vi "test - Auto Removal of Rules in CSM.vi"(8 "error in (no error)":errorcluster, 11 "TestCase in":refnum<class "testcase-Broadcast Registry.lvclass">) -> (0 "error out":errorcluster, 3 "TestCase out":refnum<class "testcase-Broadcast Registry.lvclass">)   [LabVIEW 2017, in "testcase-Broadcast Registry.lvclass"]
uses:
  testcase-Broadcast Registry.lvclass
  f1ab6f25-c30d-499f-96ca-3a55fa643449.vi
  3333bc11-4669-4098-bb8f-070e1dff9beb.vi
  src/user.lib/_NEVSTOP/Communicable State Machine(CSM)/AdvanceAPI/CSM - Revert Arguments-Safe String.vi
  src/user.lib/_NEVSTOP/Communicable State Machine(CSM)/AdvanceAPI/CSM - Make String Arguments Safe.vi
  src/user.lib/_NEVSTOP/Communicable State Machine(CSM)/AdvanceAPI/CSM - Break Down Multiple States String.vi
  src/user.lib/_NEVSTOP/Communicable State Machine(CSM)/AdvanceAPI/CSM - Compact Multiple States.vi
  src/user.lib/_NEVSTOP/Communicable State Machine(CSM)/AdvanceAPI/CSM - Keywords.vi
  src/user.lib/_NEVSTOP/Communicable State Machine(CSM)/_Shared/Trim Single-line Text.vi
  <vilib>/addons/_JKI Toolkits/VI Tester/TestCase.llb/TestCase.lvclass
  src/user.lib/_NEVSTOP/Communicable State Machine(CSM)/Communicable State Machine.lvlib
  C:/Program Files (x86)/National Instruments/LabVIEW 2017/vi.lib/addons/_JKI Toolkits/VI Tester/TestCase.llb/TestCase.lvclass
panel:
  out "Entries":T1(array[cluster])
  out "Error Occurred":errorcluster
  out "State History":string
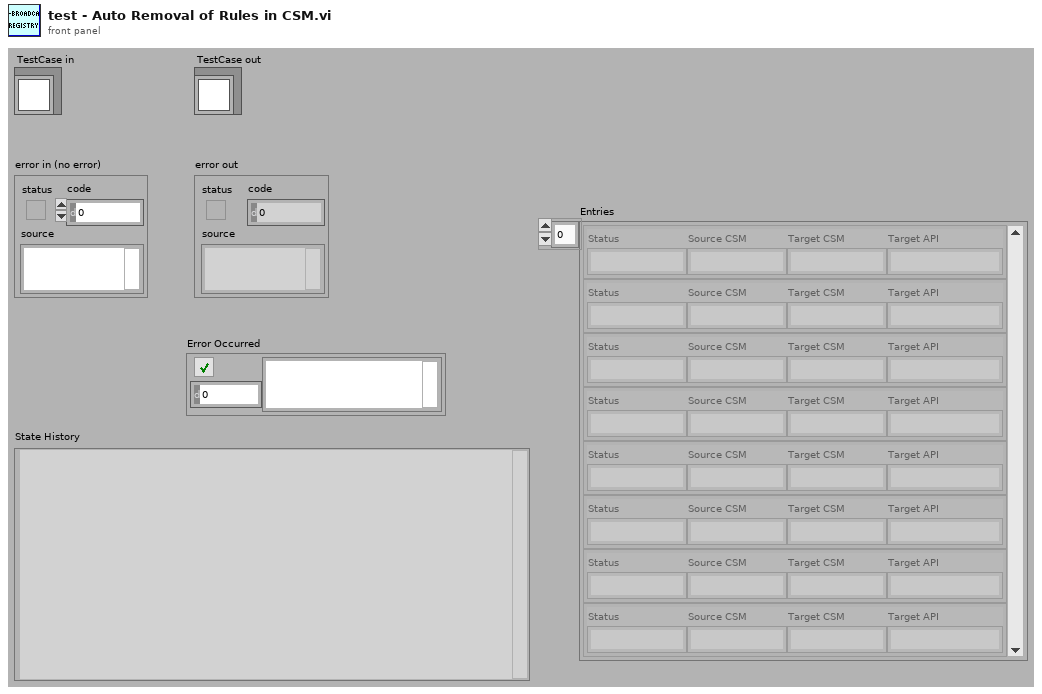
[diagram p1: front panel]
types:
  T1 = cluster{"Status":string, "Source CSM":string, "Target CSM":string, "Target API":string}[]
  T2 = enum32{"Invalid", "Standard", "Closed", "Hidden", "Minimized", "Maximized"}
  T3 = enum32{"invalid app kind", "Development System", "Run Time System", "Student Edition", "Embedded LabVIEW", "Evaluation", "Custom"}
  T4 = typedef "Communicable State Machine.lvlib/_CSM_Response Source Message.ctl" = cluster{"‘State":string, "’Arguments":string, "’Error":errorcluster}
  T5 = cluster{"Current VI Reference":refnum<vi>, "Close Panel on Exit?":bool}
  T6 = cluster{"Core":cluster{"Current VI Reference":refnum<vi>, "Close Panel on Exit?":bool}, "Your Boolean data":bool, "Your string data":string}
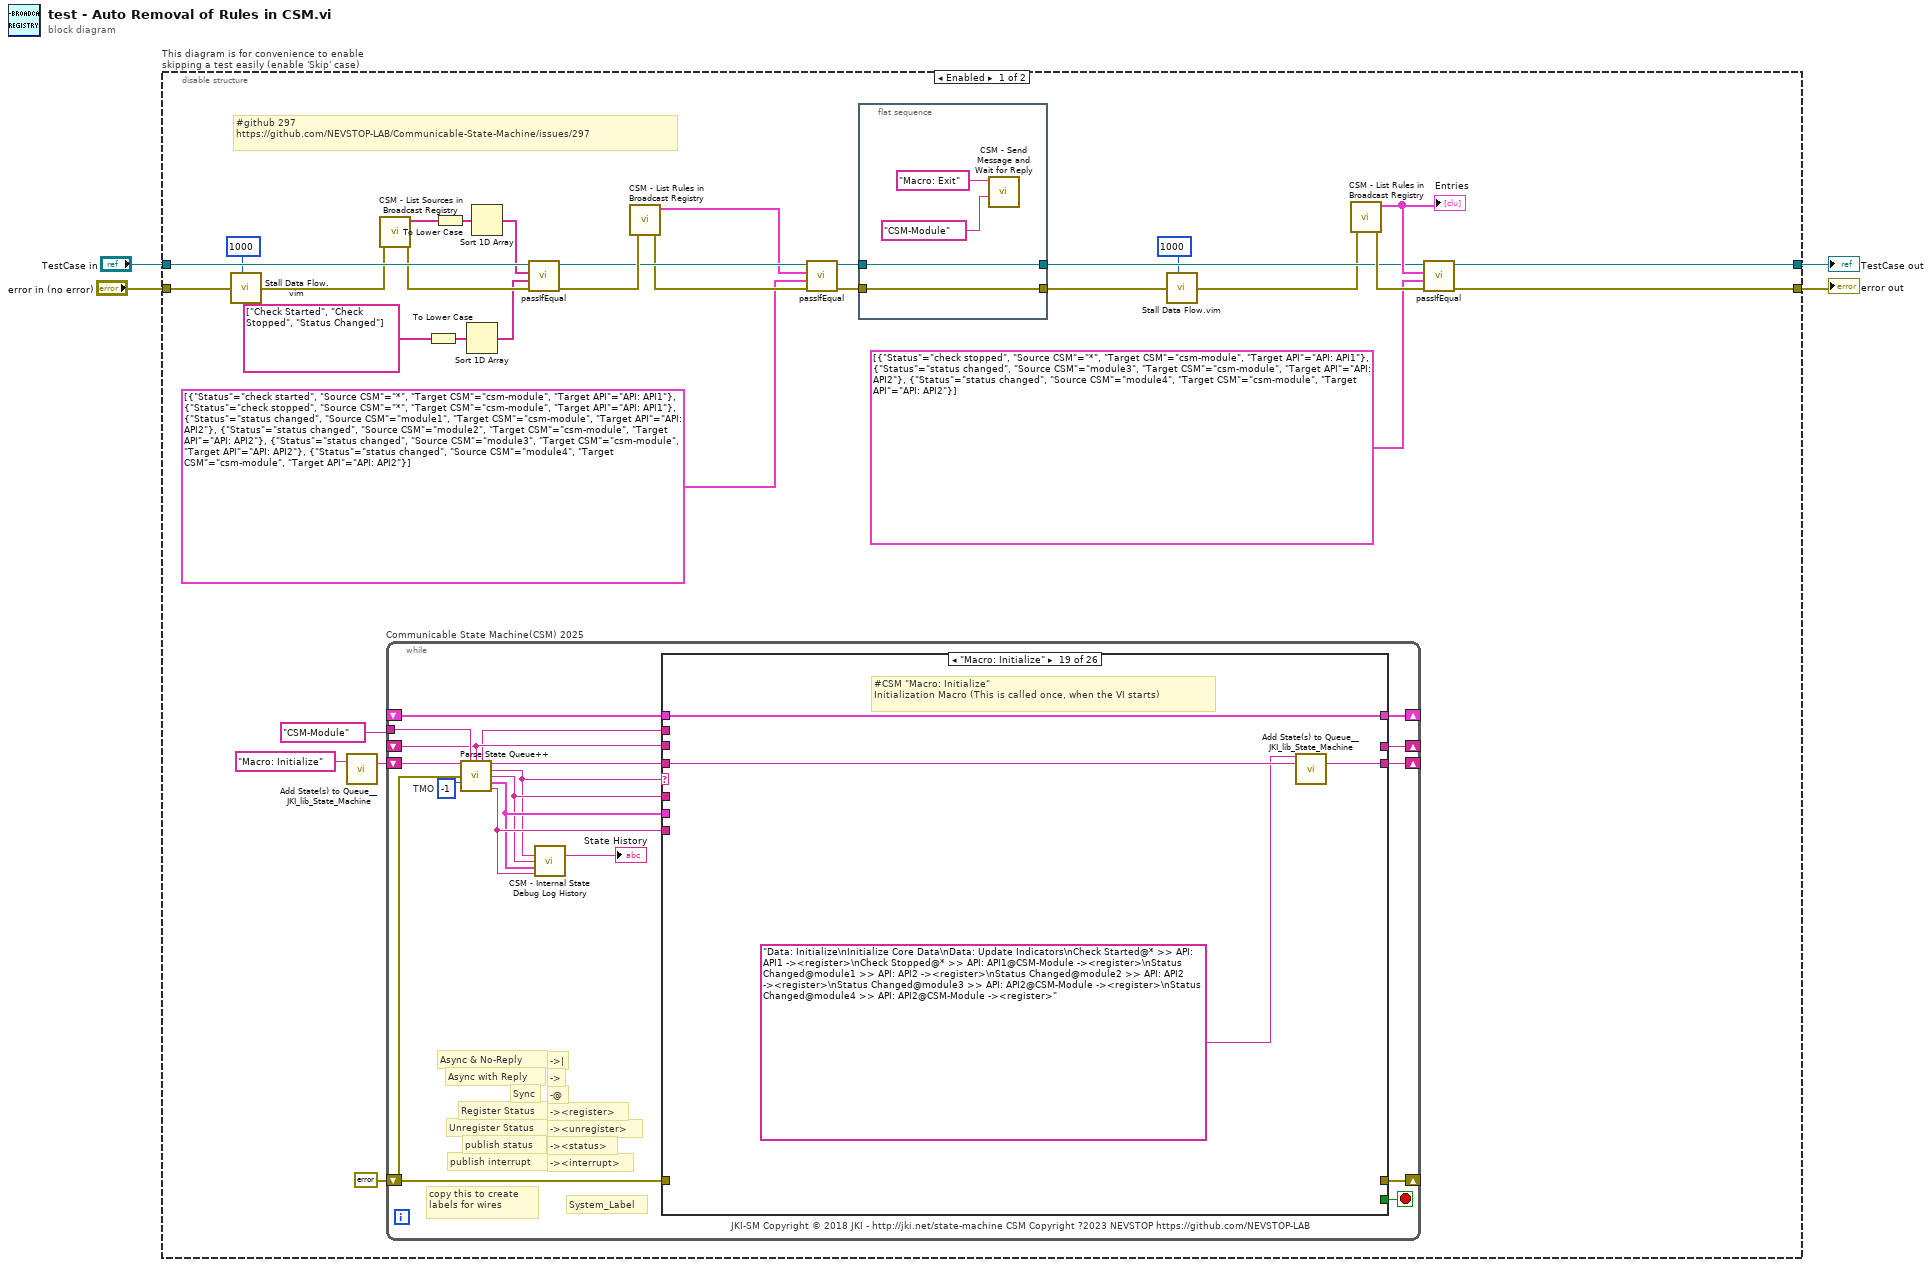
[diagram p0: block diagram]
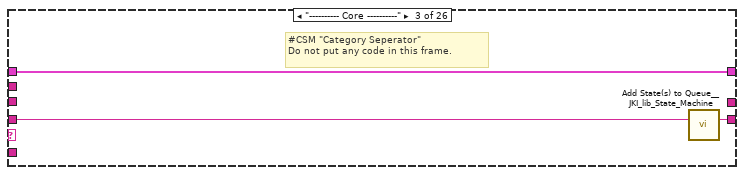
[diagram p4: hidden frame]
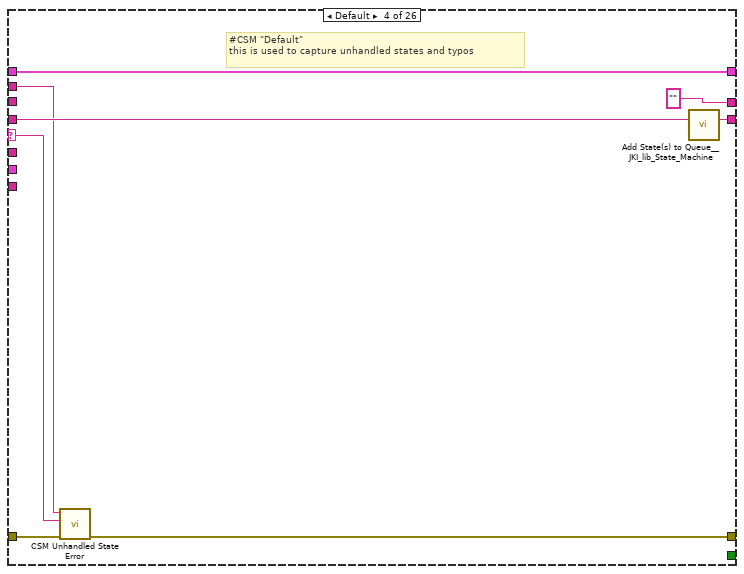
[diagram p5: hidden frame]
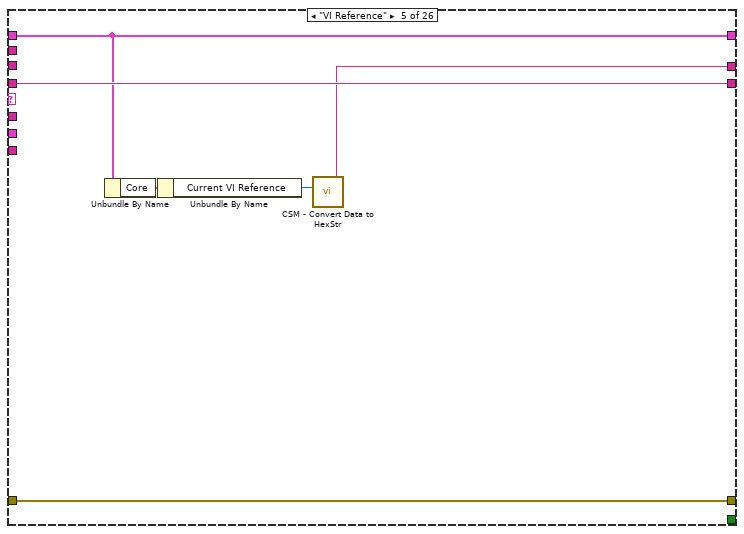
[diagram p6: hidden frame]
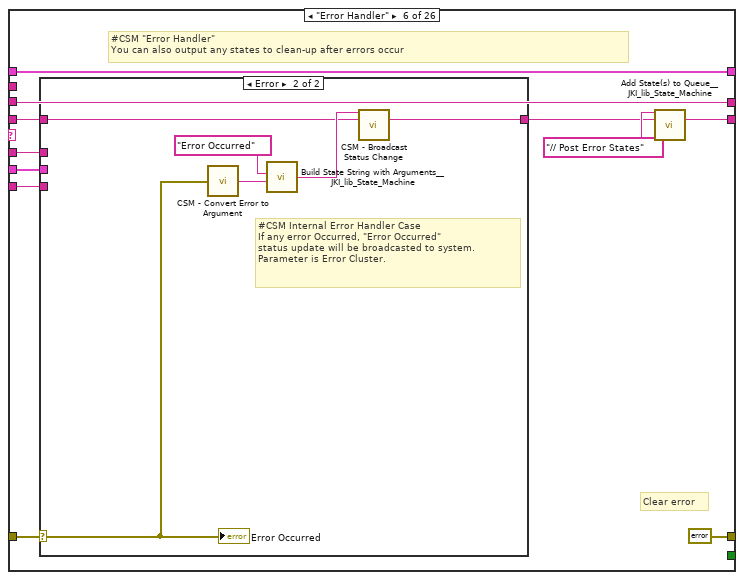
[diagram p7: hidden frame]
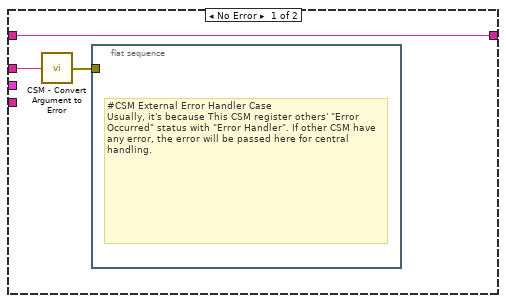
[diagram p8: hidden frame]
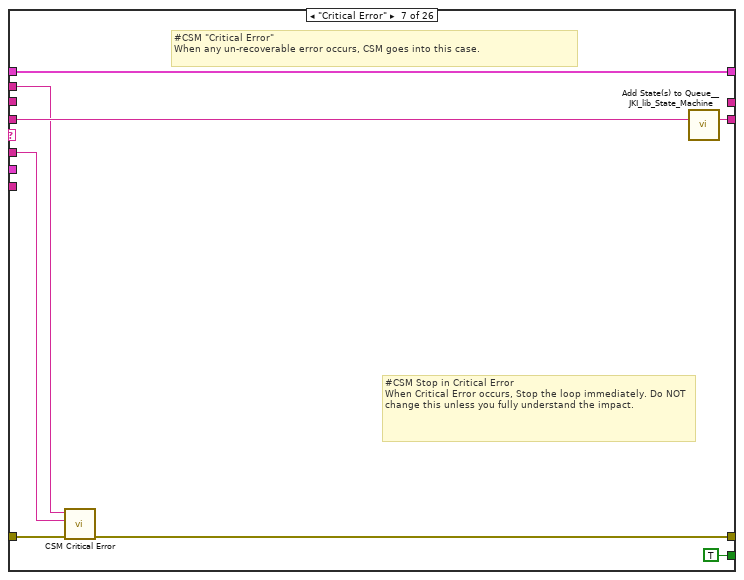
[diagram p9: hidden frame]
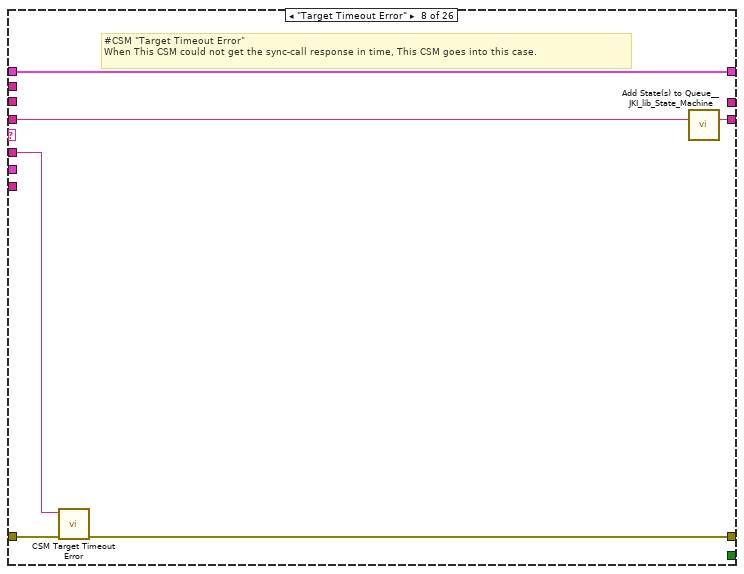
[diagram p10: hidden frame]
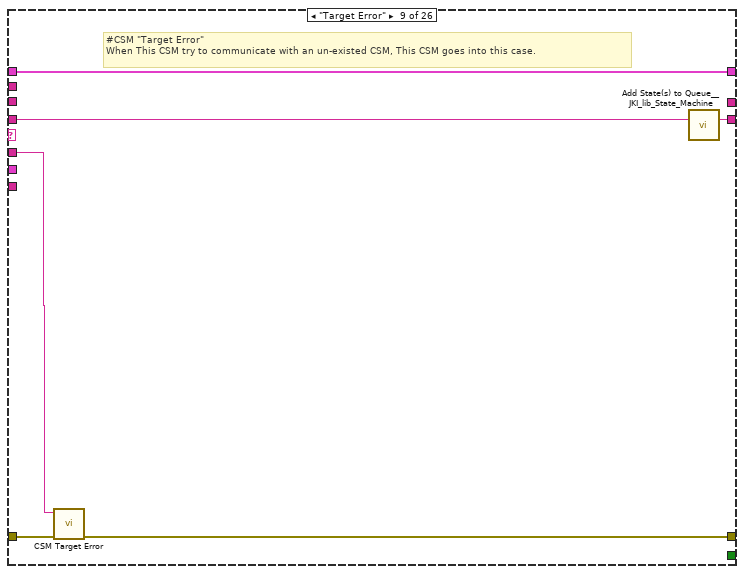
[diagram p11: hidden frame]
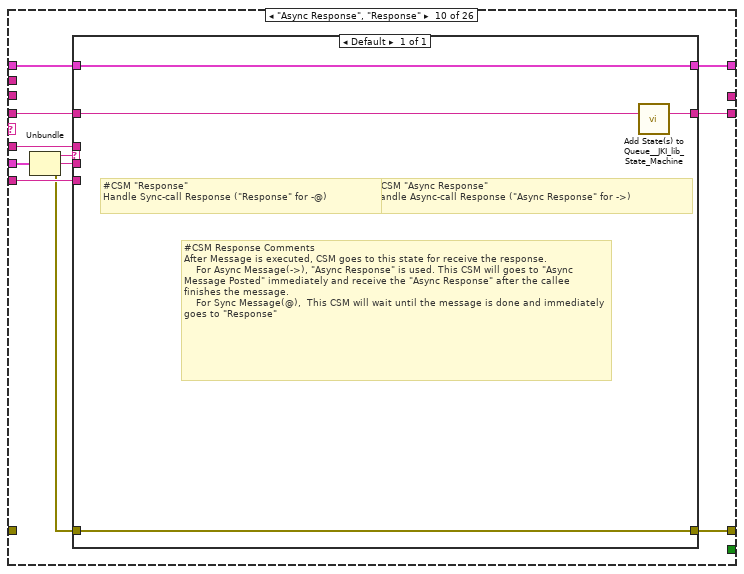
[diagram p12: hidden frame]
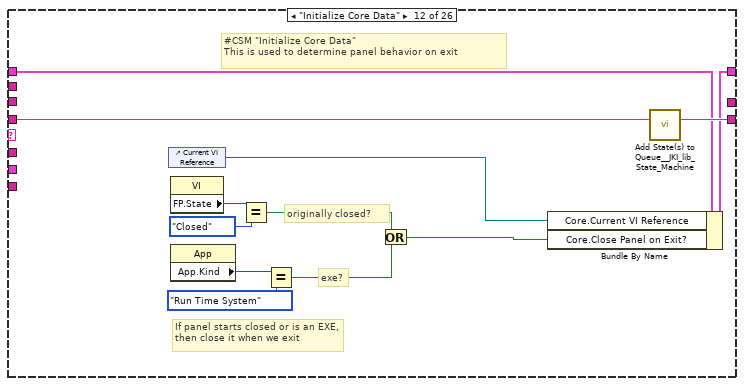
[diagram p14: hidden frame]
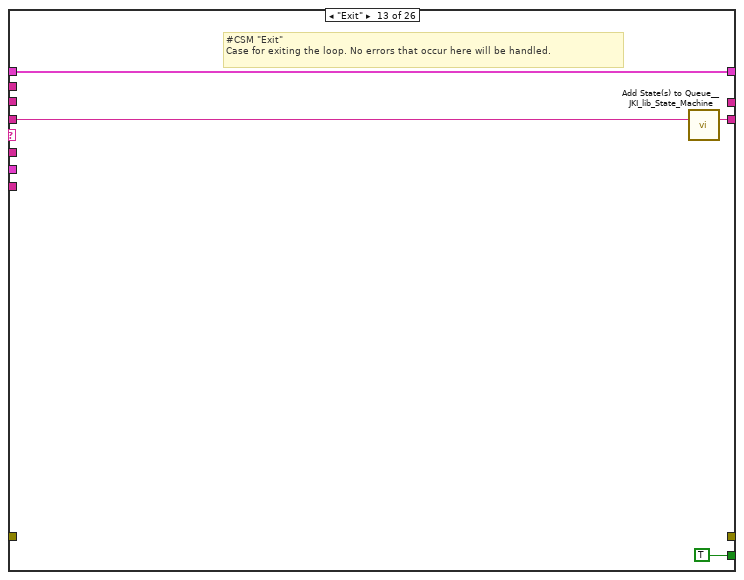
[diagram p15: hidden frame]
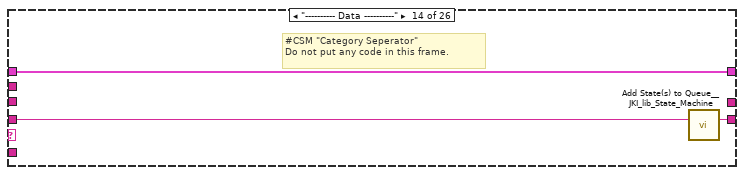
[diagram p16: hidden frame]
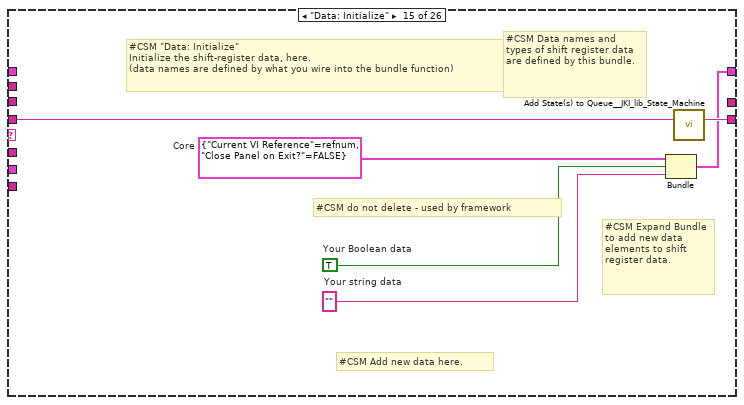
[diagram p17: hidden frame]
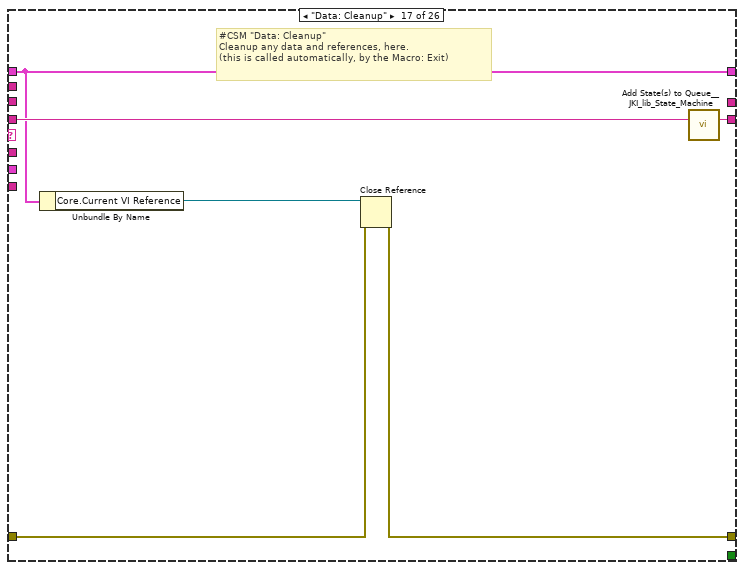
[diagram p19: hidden frame]
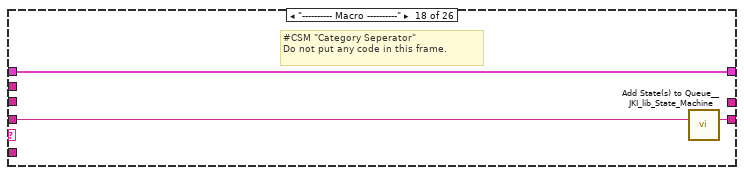
[diagram p20: hidden frame]
diagram:
  n1 = disable-structure "This diagram is for convenience to enable skipping a test easily (enable 'Skip' case)" shown="Enabled" {
    disable-tunnel: "TestCase in" -> [w35 w205]
    disable-tunnel: [w17 w203] -> w1
    disable-tunnel: [w24 w204] -> w3
    disable-tunnel: "error in (no error)" -> [w34 w202]
    frame Enabled {
      # "#github 297\nhttps://github.com/NEVSTOP-LAB/Communicable-State-Machine/issues/297"
      n2 = call "Stall Data Flow.vim"("value in"=w34, "milliseconds to wait"=u32 1000) -> ("value out"=w29:errorcluster)  [unwired: 1 out]
      n3 = call <vilib>:"Add State(s) to Queue__JKI_lib_State_Machine.vi"("State(s) in (\"\")"="Macro: Initialize" ("Init State(\"Macro: Initialize\")")) -> ("States Out"=w33:string)  [unwired: 14 in]
      n4 = call "CSM - List Sources in Broadcast Registry.vi"("error in (no error)"=w29) -> ("error out"=w27:errorcluster, "Broadcast Names"=w26:string[])  [unwired: 9 in]
      n5 = while "Communicable State Machine(CSM) 2025" {
        shift-right: [w52] -> _
        shift-left: _ -> [w51]
        shift-right: [w55] -> _
        shift-left: errorcluster {"status"=FALSE, "code"=0, "source"=""} ("error out") -> [w41]
        shift-right: [w54] -> _
        shift-left: w33 -> [w56]
        tunnel: "CSM-Module" ("Name (\"\" to Use UUID)") -> [w48]
        shift-right: [w49] -> _
        shift-left: _ -> [w43]
        stop <- w53 stop-if-true
        w50 = -1  # TMO
        # "-><interrupt>"
        # "-><status>"
        # "-><unregister>"
        # "-><register>"
        # "-@"
        # "->"
        # "->|"
        # "publish interrupt"
        # "publish status"
        # "Unregister Status"
        # "Register Status"
        # "Sync"
        # "Async with Reply"
        # "Async & No-Reply"
        # "JKI-SM Copyright © 2018 JKI - http://jki.net/state-machine CSM Copyright ?2023 NEVSTOP https://github.com/NEVSTOP-LAB"
        # "copy this to create labels for wires"
        # "System_Label"
        n6 = call "Parse State Queue++.vi"("State Queue"=w56, "Name (\"\" to Use UUID)"=w48, "Response Arguments"=w43, "Previous Error"=w41, "Dequeue (1 ms)"=w50) -> ("Name Used"=w42:string, "Remaining States"=w57:string, "Current State"=w44:string, "Arguments"=w45:string, "Additional Information"=w46:T4, "Source CSM"=w47:string)  [unwired: 5 in]
        n7 = call "CSM - Internal State Debug Log History.vi"("State"=w44, "Arguments (\"\")"=w45, ">> Response Source Message >>"=w46, "Source (\"\")"=w47) -> ("Debug Log"=→"State History":string)  [unwired: 11 in]
        n8 = case shown="\"Macro: Initialize\"" w44 {
          selector: w44 -> [_ _ _ w68 _ _ _ _ _ _ _ _ _ _ _ _ _ _ _ _ _ _ _ _ _ _]
          tunnel: w57 -> [w58 w61 w64 w72 w77 w83 w106 w112 w118 w128 w135 w147 w151 w154 w160 w162 w168 w171 w175 w181 w183 w186 w190 w195 w198 w201]
          tunnel: w45 -> [_ _ _ _ _ w82 w102 w109 w115 w122 _ _ _ _ _ _ _ _ _ _ _ _ w188 _ _ _]
          tunnel: w51 -> [w59 w60 w62 w70 w76 w88 w104 w110 w116 w126 w134 w141 w149 w152 _ w161 w163 w169 w173 w179 w182 w185 w189 w193 w196 w199]
          tunnel: [_ _ _ w65 w78 errorcluster {"status"=FALSE, "code"=0, "source"=""} ("error out") w99 w107 w113 w129 _ _ _ _ _ _ w164 _ _ _ _ _ _ _ _ _] -> w55
          tunnel: w41 -> [_ _ _ w66 w78 w86 w100 w108 w114 _ _ _ _ _ _ _ w165 _ _ _ _ _ _ _ _ _]
          tunnel: [w58 w61 w63 w71 w77 w84 w105 w111 w117 w127 w135 w146 w150 w153 w159 w162 w167 w170 w174 w180 w183 w186 w190 w194 w197 w200] -> w54
          tunnel: [_ _ _ _ _ _ TRUE _ _ _ _ _ TRUE _ _ _ _ _ _ _ _ _ _ _ _ _] -> w53
          tunnel: [w59 w60 w62 w70 w76 w88 w104 w110 w116 w125 w134 w145 w149 w152 w158 w161 w163 w169 w173 w179 w182 w185 w189 w193 w196 w199] -> w52
          tunnel: w47 -> [_ _ _ _ _ w81 _ _ _ w123 _ _ _ _ _ _ _ _ _ _ _ _ _ _ _ _]
          tunnel: w46 -> [_ _ _ _ _ w80 _ _ _ w124 _ _ _ _ _ _ _ _ _ _ _ _ _ _ _ _]
          tunnel: [_ _ _ "" w73 w79 _ _ _ _ _ _ _ _ _ _ _ _ _ _ _ "API1 Response" w187 _ _ _] -> w49
          tunnel: w42 -> [_ _ _ w67 _ _ w101 _ _ _ _ _ _ _ _ _ _ _ _ _ _ _ _ _ _ _]
          tunnel: w43 -> [_ _ _ _ _ w79 _ _ _ _ _ _ _ _ _ _ _ _ _ _ _ _ _ _ _ _]
          frame "", "Idle" {
            # "#CSM \"Idle/Event Handler\"\nexecutes when the state queue is empty"
          }
          frame "CSM Documentation" {
            # "#CSM Documentation"
            # "#CSM State Syntax\n\n// Comment line, all text to the right of “//” will be ignored\n// Local Message Example\nDoSth: DoA >> Arguments\n\n// Sync Call Example\nAPI: xxxx >> Arguments -@ TargetModule\n\n// Async Call Example\nAPI: xxxx >> Arguments -> TargetModule\n\n// Async Call without Reply Example\nAPI: xxxx >> Arguments ->| TargetModule\n\n// Broadcast normal status:\nStatus >> StatusArguments  -><status>\n\n// Broadcast Interrupt status:\nInterrupt >> StatusArguments  -><interrupt>\n\n// Register Source Module's status to Handler Module\nStatus@Source Module >> Handler Module@Handler Module -><register>\n\n// Unegister Source Module's status\nStatus@Source Module >> Handler Module -><unregister>"
            # "#CSM README FIRST\n\nCommunicable State Machine(CSM) is a LabVIEW application framework that builds upon JKI State Machine(JKISM). It follows the pattern of JKISM and extends the keywords to describe message communication between modules, including concepts such as Sync-Message, Async-Message, Subscription/Unsubscription of status - essential elements for creating reusable code modules. For more information, please visit the CSM wiki: https://nevstop-lab.github.io/CSM-Wiki/\n\nFor instructions on JKI State Machine, visit: \n    http://jki.net/state-machine/\nFor information about CSM, visit: \n    https://github.com/NEVSTOP-LAB"
            # "#CSM \"Documentation\"\nCase for holding CSM Documenation"
          }
          frame "---------- Core ----------" {
            # "#CSM \"Category Seperator\"\nDo not put any code in this frame."
            n9 = call <vilib>:"Add State(s) to Queue__JKI_lib_State_Machine.vi"("State(s) in (\"\")"=w64) -> ("States Out"=w63:string)  [unwired: 14 in]
          }
          frame Default {
            # "#CSM \"Default\"\nthis is used to capture unhandled states and typos"
            n10 = call "CSM Unhandled State Error.vi"("error in (no error)"=w66, "Undefined State"=w68, "CSM Name"=w67) -> ("error out"=w65:errorcluster)  [unwired: 8 in]
            n11 = call <vilib>:"Add State(s) to Queue__JKI_lib_State_Machine.vi"("State(s) in (\"\")"=w72) -> ("States Out"=w71:string)  [unwired: 14 in]
          }
          frame "VI Reference" {
            n12 = Unbundle By Name(w76) -> ("Core"=w75:T5)
            n13 = Unbundle By Name(w75) -> ("Current VI Reference"=w74:refnum<vi>)
            n14 = call "CSM - Convert Data to HexStr.vi"("Variant"=w74) -> ("HEX String (0-9,A-F)"=w73:string)  [unwired: 8 in]
          }
          frame "Error Handler" {
            # "#CSM \"Error Handler\"\nYou can also output any states to clean-up after errors occur"
            # "Clear error"
            n15 = case shown="Error" w86 {
              selector: w86 -> [_ w93]
              tunnel: [w92 w95] -> w85
              tunnel: w83 -> [w92 w94]
              tunnel: w82 -> [w91 _]
              tunnel: w81 -> [_ _]
              tunnel: w80 -> [_ _]
              frame No Error {
                n16 = call "CSM - Convert Argument to Error.vi"("Argument"=w91) -> ("Error"=w90:errorcluster)  [unwired: 4 in]
                n17 = flat-sequence {
                  tunnel: w90 -> [_]
                  frame #0 {
                    # "#CSM External Error Handler Case\nUsually, it's because This CSM register others' \"Error Occurred\" status with \"Error Handler\". If other CSM have any error, the error will be passed here for central handling."
                  }
                }
              }
              frame Error {
                # "#CSM Internal Error Handler Case \nIf any error Occurred, \"Error Occurred\" \nstatus update will be broadcasted to system.\nParameter is Error Cluster."
                n18 = call "CSM - Convert Error to Argument.vi"("Error"=w93) -> ("Argument"=w97:string)  [unwired: 4 in]
                n19 = call <vilib>:"Build State String with Arguments__JKI_lib_State_Machine.vi"("Arguments (\"\")"=w97, "State"="Error Occurred" ("Status with Arguments")) -> ("State with Arguments"=w96:string)  [unwired: 4 in]
                n20 = call "CSM - Broadcast Status Change.vi"("Status With Arguments"=w96, "State Queue"=w94) -> ("Remaining States"=w95:string)  [unwired: 13 in]
                "Error Occurred" <- w93
              }
            }
            n21 = call <vilib>:"Add State(s) to Queue__JKI_lib_State_Machine.vi"("State(s) in Front (\"\")"="// Post Error States", "State(s) in (\"\")"=w85) -> ("States Out"=w84:string)  [unwired: 13 in]
          }
          frame "Critical Error" {
            # "#CSM \"Critical Error\"\nWhen any un-recoverable error occurs, CSM goes into this case."
            # "#CSM Stop in Critical Error\nWhen Critical Error occurs, Stop the loop immediately. Do NOT change this unless you fully understand the impact."
            n22 = call "CSM Critical Error.vi"("error in (no error)"=w100, "Arugments (As Reason)"=w102, "CSM Name"=w101) -> ("error out"=w99:errorcluster)  [unwired: 8 in]
            n23 = call <vilib>:"Add State(s) to Queue__JKI_lib_State_Machine.vi"("State(s) in (\"\")"=w106) -> ("States Out"=w105:string)  [unwired: 14 in]
          }
          frame "Target Timeout Error" {
            # "#CSM \"Target Timeout Error\"\nWhen This CSM could not get the sync-call response in time, This CSM goes into this case."
            n24 = call "CSM Target Timeout Error.vi"("error in (no error)"=w108, "Arguments (As CSM Name)"=w109) -> ("error out"=w107:errorcluster)  [unwired: 9 in]
            n25 = call <vilib>:"Add State(s) to Queue__JKI_lib_State_Machine.vi"("State(s) in (\"\")"=w112) -> ("States Out"=w111:string)  [unwired: 14 in]
          }
          frame "Target Error" {
            # "#CSM \"Target Error\"\nWhen This CSM try to communicate with an un-existed CSM, This CSM goes into this case."
            n26 = call "CSM Target Error.vi"("error in (no error)"=w114, "Arguments (As CSM Name)"=w115) -> ("error out"=w113:errorcluster)  [unwired: 9 in]
            n27 = call <vilib>:"Add State(s) to Queue__JKI_lib_State_Machine.vi"("State(s) in (\"\")"=w118) -> ("States Out"=w117:string)  [unwired: 14 in]
          }
          frame "Async Response", "Response" {
            n28 = Unbundle(w124) -> ("‘State"=w121:string, "’Arguments"=w120:string, "’Error"=w119:errorcluster)
            n29 = case shown="Default" w121 {
              tunnel: [w130] -> w127
              tunnel: w128 -> [w131]
              tunnel: [w133] -> w125
              tunnel: w126 -> [w133]
              tunnel: [w132] -> w129
              tunnel: w119 -> [w132]
              tunnel: w123 -> [_]
              tunnel: w122 -> [_]
              tunnel: w120 -> [_]
              frame Default {
                # "#CSM \"Async Response\"\nHandle Async-call Response (\"Async Response\" for ->)"
                # "#CSM \"Response\"\nHandle Sync-call Response (\"Response\" for -@)"
                # "#CSM Response Comments\nAfter Message is executed, CSM goes to this state for receive the response.\n    For Async Message(->), \"Async Response\" is used. This CSM will goes to \"Async Message Posted\" immediately and receive the \"Async Response\" after the callee finishes the message.\n    For Sync Message(@),  This CSM will wait until the message is done and immediately goes to \"Response\""
                n30 = call <vilib>:"Add State(s) to Queue__JKI_lib_State_Machine.vi"("State(s) in (\"\")"=w131) -> ("States Out"=w130:string)  [unwired: 14 in]
              }
            }
          }
          frame "Async Message Posted" {
            # "#CSM \"Async Message Posted\"\nAfter Async Message is posted (-> or ->| ), CSM goes to this state for post-action.\nYou can use Argument - State to tell which Async Message is called."
          }
          frame "Initialize Core Data" {
            # "#CSM \"Initialize Core Data\"\nThis is used to determine panel behavior on exit"
            # "originally closed?"
            # "exe?"
            # "If panel starts closed or is an EXE, then close it when we exit"
            n31 = control-ref of="Current VI Reference"() -> (w139:refnum<vi>)
            n32 = property class="VI"() -> ("FP.State"=w138:T2)  [unwired: 2 in, 2 out]
            n33 = property class="App"() -> ("App.Kind"=w144:T3)  [unwired: 2 in, 2 out]
            n34 = Equal?(x=w138, y=T2."Closed" ("Front Panel Window:State")) -> (x = y?=w136:bool)
            n35 = Equal?(x=w144, y=T3."Run Time System" ("Application:Kind")) -> (x = y?=w142:bool)
            n36 = Or(x=w136, y=w142) -> (x .or. y?=w140:bool)
            n37 = Bundle By Name(cluster=w141, "Core.Current VI Reference"=w139, "Core.Close Panel on Exit?"=w140) -> (w145:T6)
            n38 = call <vilib>:"Add State(s) to Queue__JKI_lib_State_Machine.vi"("State(s) in (\"\")"=w147) -> ("States Out"=w146:string)  [unwired: 14 in]
          }
          frame "Exit" {
            # "#CSM \"Exit\"\nCase for exiting the loop. No errors that occur here will be handled."
            n39 = call <vilib>:"Add State(s) to Queue__JKI_lib_State_Machine.vi"("State(s) in (\"\")"=w151) -> ("States Out"=w150:string)  [unwired: 14 in]
          }
          frame "---------- Data ----------" {
            # "#CSM \"Category Seperator\"\nDo not put any code in this frame."
            n40 = call <vilib>:"Add State(s) to Queue__JKI_lib_State_Machine.vi"("State(s) in (\"\")"=w154) -> ("States Out"=w153:string)  [unwired: 14 in]
          }
          frame "Data: Initialize" {
            w155 = T5 {"Current VI Reference"=refnum, "Close Panel on Exit?"=FALSE}  # Core
            w157 = TRUE  # Your Boolean data
            w156 = ""  # Your string data
            # "#CSM \"Data: Initialize\"\nInitialize the shift-register data, here.\n(data names are defined by what you wire into the bundle function)"
            # "#CSM do not delete - used by framework"
            # "#CSM Expand Bundle to add new data elements to shift register data."
            # "#CSM Add new data here."
            # "#CSM Data names and types of shift register data are defined by this bundle."
            n41 = Bundle("Core"=w155, "Your Boolean data"=w157, "Your string data"=w156) -> (w158:T6)  [unwired: 1 in]
            n42 = call <vilib>:"Add State(s) to Queue__JKI_lib_State_Machine.vi"("State(s) in (\"\")"=w160) -> ("States Out"=w159:string)  [unwired: 14 in]
          }
          frame "Data: Update Indicators" {
          }
          frame "Data: Cleanup" {
            # "#CSM \"Data: Cleanup\"\nCleanup any data and references, here.\n(this is called automatically, by the Macro: Exit)"
            n43 = Unbundle By Name(w163) -> ("Core.Current VI Reference"=w166:refnum<vi>)
            n44 = Close Reference(reference=w166, error in (no error)=w165) -> (error out=w164:errorcluster)
            n45 = call <vilib>:"Add State(s) to Queue__JKI_lib_State_Machine.vi"("State(s) in (\"\")"=w168) -> ("States Out"=w167:string)  [unwired: 14 in]
          }
          frame "---------- Macro ----------" {
            # "#CSM \"Category Seperator\"\nDo not put any code in this frame."
            n46 = call <vilib>:"Add State(s) to Queue__JKI_lib_State_Machine.vi"("State(s) in (\"\")"=w171) -> ("States Out"=w170:string)  [unwired: 14 in]
          }
          frame "Macro: Initialize" {
            # "#CSM \"Macro: Initialize\"\nInitialization Macro (This is called once, when the VI starts)"
            n47 = call <vilib>:"Add State(s) to Queue__JKI_lib_State_Machine.vi"("State(s) in Front (\"\")"="Data: Initialize\nInitialize Core Data\nData: Update Indicators\nCheck Started@* >> API: API1 -><register>\nCheck Stopped@* >> API: API1@CSM-Module -><register>\nStatus Changed@module1 >> API: API2 -><register>\nStatus Changed@module2 >> API: API2 -><register>\nStatus Changed@module3 >> API: API2@CSM-Module -><register>\nStatus Changed@module4 >> API: API2@CSM-Module -><register>", "State(s) in (\"\")"=w175) -> ("States Out"=w174:string)  [unwired: 13 in]
          }
          frame "Macro: Exit" {
            # "#CSM \"Macro: Exit\"\nExit Macro (This is called once, when the VI exits)"
            n48 = call <vilib>:"Add State(s) to Queue__JKI_lib_State_Machine.vi"("State(s) in Front (\"\")"="//Exit Sub-Modules ", "State(s) at Back (\"\")"="Data: Cleanup\nExit") -> ("States Out"=w177:string)  [unwired: 13 in]
            n49 = call <vilib>:"Add State(s) to Queue__JKI_lib_State_Machine.vi"("State(s) in Front (\"\")"=w177, "State(s) in (\"\")"=w181) -> ("States Out"=w180:string)  [unwired: 13 in]
          }
          frame "---------- API ----------" {
            # "#CSM \"Category Seperator\"\nDo not put any code in this frame."
          }
          frame "API: API1" {
            # "#CSM API Example\nCopy/Rename this case for your own API"
            # "#CSM >> Msg/Rep's CSM >>\nIf you need to tell who triggered this state , use this string. If it's this case itself, this string is \"\"."
            # "#CSM >> Arguments >>\nDeal with the parameter if any"
            # "#CSM Response\nConnect this to return the response of your API"
          }
          frame "API: API2" {
            # "#CSM API Example\nCopy/Rename this case for your own API"
            # "unpack Hex String  to Variant\nif complex parameter is needed."
            n50 = call "CSM - Convert HexStr to Data.vi"("HEX String"=w188) -> ()  [unwired: 7 in, 2 out]
            n51 = disable-structure shown="Disabled" {
              disable-tunnel: [w191 "API2 Response"] -> w187
              frame Disabled {
                # "pack variant to hexstr \nif complex response is needed."
                # "complex Response"
                n52 = call "CSM - Convert Data to HexStr.vi"() -> ("HEX String (0-9,A-F)"=w191:string)  [unwired: 9 in]
              }
              frame Enabled {
              }
            }
          }
          frame "---------- Action ----------" {
            # "#CSM \"Category Seperator\"\nDo not put any code in this frame."
            n53 = call <vilib>:"Add State(s) to Queue__JKI_lib_State_Machine.vi"("State(s) in (\"\")"=w195) -> ("States Out"=w194:string)  [unwired: 14 in]
          }
          frame "Action: action1" {
            # "#CSM \"Internal State\"\nThis category is used for holding internal states"
            n54 = call <vilib>:"Add State(s) to Queue__JKI_lib_State_Machine.vi"("State(s) in (\"\")"=w198) -> ("States Out"=w197:string)  [unwired: 14 in]
          }
          frame "Action: action2" {
            # "#CSM \"Internal State\"\nThis category is used for holding internal states"
            n55 = call <vilib>:"Add State(s) to Queue__JKI_lib_State_Machine.vi"("State(s) in (\"\")"=w201) -> ("States Out"=w200:string)  [unwired: 14 in]
          }
        }
      }
      n56 = To Lower Case(string=string[] ["Check Started", "Check Stopped", "Status Changed"] ("Status in Registry")) -> (all lower case string=w21:string[])
      n57 = To Lower Case(string=w26) -> (all lower case string=w20:string[])
      n58 = Sort 1D Array(array=w21) -> (sorted array=w22:string[])
      n59 = Sort 1D Array(array=w20) -> (sorted array=w23:string[])
      n60 = call-dynamic "passIfEqual.vi"("error in (no error)"=w27, "y"=w22, "x"=w23, "TestCase in"=w35) -> ("error out"=w19:errorcluster, "TestCase out"=w18:refnum<class "testcase-Broadcast Registry.lvclass">)  [unwired: 6 in]
      n61 = call "CSM - List Rules in Broadcast Registry.vi"("error in (no error)"=w19) -> ("error out"=w16:errorcluster, "Rule Entries"=w15:T1)  [unwired: 9 in]
      n62 = call-dynamic "passIfEqual.vi"("error in (no error)"=w16, "y"=T1 [{"Status"="check started", "Source CSM"="*", "Target CSM"="csm-module", "Target API"="API: API1"}, {"Status"="check stopped", "Source CSM"="*", "Target CSM"="csm-module", "Target API"="API: API1"}, {"Status"="status changed", "Source CSM"="module1", "Target CSM"="csm-module", "Target API"="API: API2"}, {"Status"="status changed", "Source CSM"="module2", "Target CSM"="csm-module", "Target API"="API: API2"}, {"Status"="status changed", "Source CSM"="module3", "Target CSM"="csm-module", "Target API"="API: API2"}, {"Status"="status changed", "Source CSM"="module4", "Target CSM"="csm-module", "Target API"="API: API2"}] ("Entries"), "x"=w15, "TestCase in"=w18) -> ("error out"=w10:errorcluster, "TestCase out"=w11:refnum<class "testcase-Broadcast Registry.lvclass">)  [unwired: 6 in]
      n63 = flat-sequence {
        tunnel: [w37] -> w9
        tunnel: w10 -> [w37]
        tunnel: [w36] -> w8
        tunnel: w11 -> [w36]
        frame #0 {
          n64 = call "CSM - Send Message and Wait for Reply.vi"("Target Module"="CSM-Module" ("Name (\"\" to Use UUID)"), "State"="Macro: Exit") -> ()  [unwired: 7 in, 3 out]
        }
      }
      n65 = call "Stall Data Flow.vim"("value in"=w9, "milliseconds to wait"=u32 1000) -> ("value out"=w6:errorcluster)  [unwired: 1 out]
      n66 = call "CSM - List Rules in Broadcast Registry.vi"("error in (no error)"=w6) -> ("error out"=w14:errorcluster, "Rule Entries"=w13:T1)  [unwired: 9 in]
      "Entries" <- w13
      n67 = call-dynamic "passIfEqual.vi"("error in (no error)"=w14, "y"=T1 [{"Status"="check stopped", "Source CSM"="*", "Target CSM"="csm-module", "Target API"="API: API1"}, {"Status"="status changed", "Source CSM"="module3", "Target CSM"="csm-module", "Target API"="API: API2"}, {"Status"="status changed", "Source CSM"="module4", "Target CSM"="csm-module", "Target API"="API: API2"}] ("Entries"), "x"=w13, "TestCase in"=w8) -> ("error out"=w24:errorcluster, "TestCase out"=w17:refnum<class "testcase-Broadcast Registry.lvclass">)  [unwired: 6 in]
    }
    frame Disabled {
      # "skip test result while test is under development"
      n68 = call <vilib>:"skip.vi"("error in (no error)"=w202, "TestCase in"=w205) -> ("error out"=w204:errorcluster, "TestCase out"=w203:refnum<class "testcase-Broadcast Registry.lvclass">)  [unwired: 8 in]
    }
  }
  "error out" <- w3
  "TestCase out" <- w1
